vi "Clear.vi"(8 "error in (no error)":errorcluster, 11 "Process In":refnum<class "Broadcast Message Receiver.lvclass">) -> (0 "error out":errorcluster)   [LabVIEW 2020, in "Broadcast Message Receiver.lvclass"]
doc: "Clears any resorces allocated during initialization."
uses:
  Broadcast Message Receiver.lvclass
  Broadcast Message Receiver.lvclass/Broadcast Message Receiver.ctl
  Process/Debug Process.lvclass
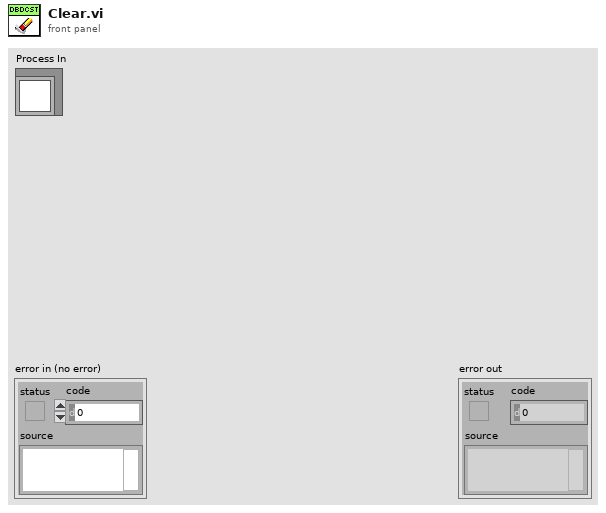
[diagram p1: front panel]
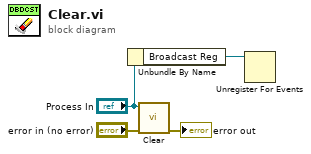
[diagram p0: block diagram]
diagram:
  n1 = Unbundle By Name("Process In") -> ("Broadcast Reg"=w1:refnum<event-registration>)
  n2 = call-parent "Clear.vi"("error in (no error)"="error in (no error)", "Process In"="Process In") -> ("error out"=→"error out":errorcluster)  [unwired: 9 in]
  n3 = Unregister For Events(event registration refnum=w1) -> ()  [unwired: 1 in, 1 out]
